vi "File Action V1.vi"(0 "Action":string, 2 "Mode":u16(ring) items=["Read", "Write"], 7 "Image Acquisition Parameters":T2={"Scan Type"=enum."Sample Scanning", "Scan Mode"=enum."XY", "Fast Axis Frequency (Hz)"=100.0, "Image Format"=128, "Line Accumulations"=1, "Frames Per Capture"=1, "Frames Accumulations"=1, "Image Dimension (um)"=[], "Number of Z Steps"=1, "Z Steps Size (um)"=1.0, "Pixel Size (nm)"=[], "Customized Image Format"=[]} {"Z Steps Size (um)" min=0.0; "Number of Z Steps" min=1; "Frames Accumulations" min=1; "Frames Per Capture" min=1; "Line Accumulations" min=1; "Image Format" items=["64 x 64"=64, "128 x 128"=128, "256 x 256"=256, "512 x 512"=512, "1024 x 1024"=1024, "2048 x 2048"=2048, "Customized..."=0]}, 9 "Manual Controls In":T1={"Galvo 1 Position (I16)"=-280, "Galvo 2 Position (I16)"=0, "X Axis Voltage (I16)"=0, "Y Axis Voltage (I16)"=0, "Z Axis Voltage (I16)"=0, "Res Mirror Amp (I16)"=0, "Res Mirror Mute"=FALSE, "Upper Shutter"=FALSE, "Lower Shutter"=FALSE}, 11 "File Path IN":path, 13 "Number of Channels":i32) -> (4 "File Path OUT":path, 8 "File REFs":refnum<file>[](array[refnum]), 15 "Files Open":bool)   [LabVIEW 2014]
uses:
  Type Defs/Image Acquisition Parameters.ctl
  Manual Controls V2.ctl
panel:
  # "Length"
  # "Height"
  # "XY"
  # "Z"
  # "Length"
  # "Height"
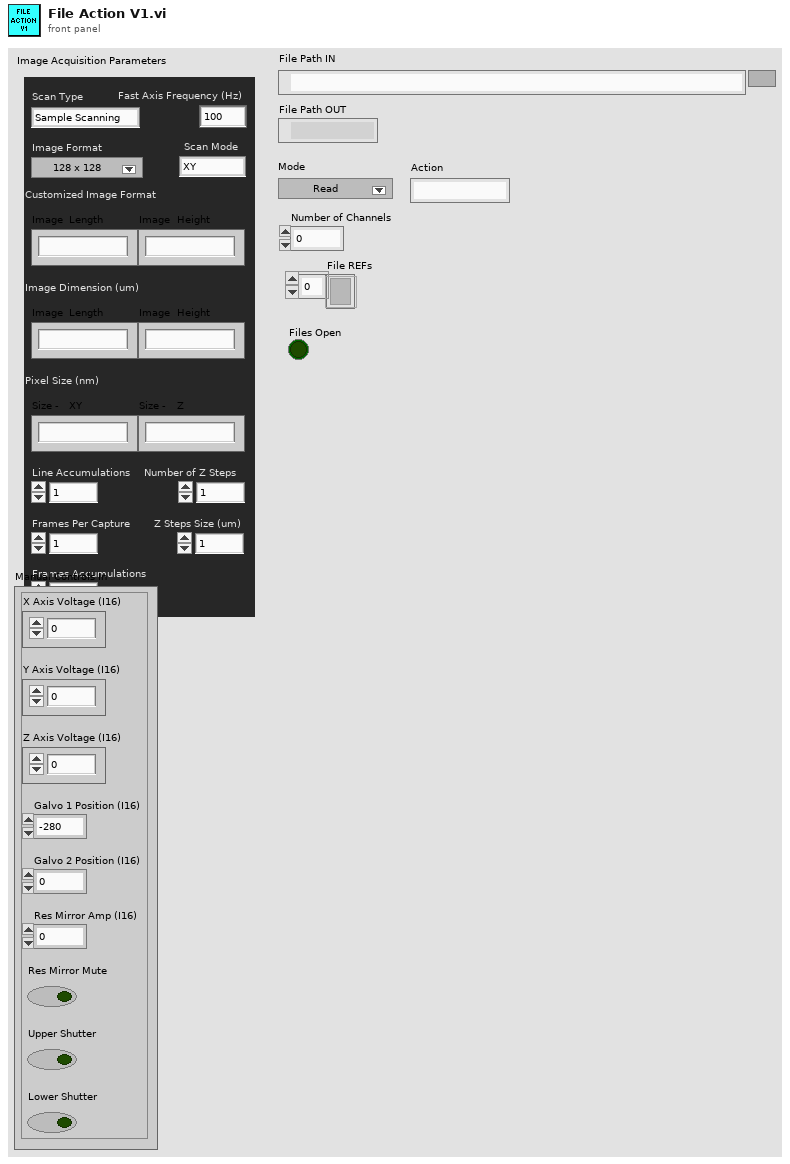
[diagram p1: front panel]
types:
  T1 = typedef "Manual Controls V2.ctl" = cluster{"Galvo 1 Position (I16)":i16, "Galvo 2 Position (I16)":i16, "X Axis Voltage (I16)":i16, "Y Axis Voltage (I16)":i16, "Z Axis Voltage (I16)":i16, "Res Mirror Amp (I16)":i16, "Res Mirror Mute":bool, "Upper Shutter":bool, "Lower Shutter":bool}
  T2 = typedef "Image Acquisition Parameters.ctl" = cluster{"Scan Type":enum16{"Sample Scanning", "Beam Scanning"}, "Scan Mode":enum16{"XY", "XZ", "YZ", "XYZ"}, "Fast Axis Frequency (Hz)":dbl, "Image Format":u16, "Line Accumulations":u16, "Frames Per Capture":u16, "Frames Accumulations":u16, "Image Dimension (um)":dbl[], "Number of Z Steps":u16, "Z Steps Size (um)":dbl, "Pixel Size (nm)":dbl[], "Customized Image Format":dbl[]}
  T3 = cluster{"Z Length (um)":sgl, "Y Length (um)":sgl, "X Length (um)":sgl, "t (s)":sgl}
  T4 = cluster{"Upper Shutter":bool, "Lower Shutter":bool}
  T5 = cluster{"Number of Z Steps":u16, "Image Format":u16, "Image Format":u16, "Frames Per Capture":u16}
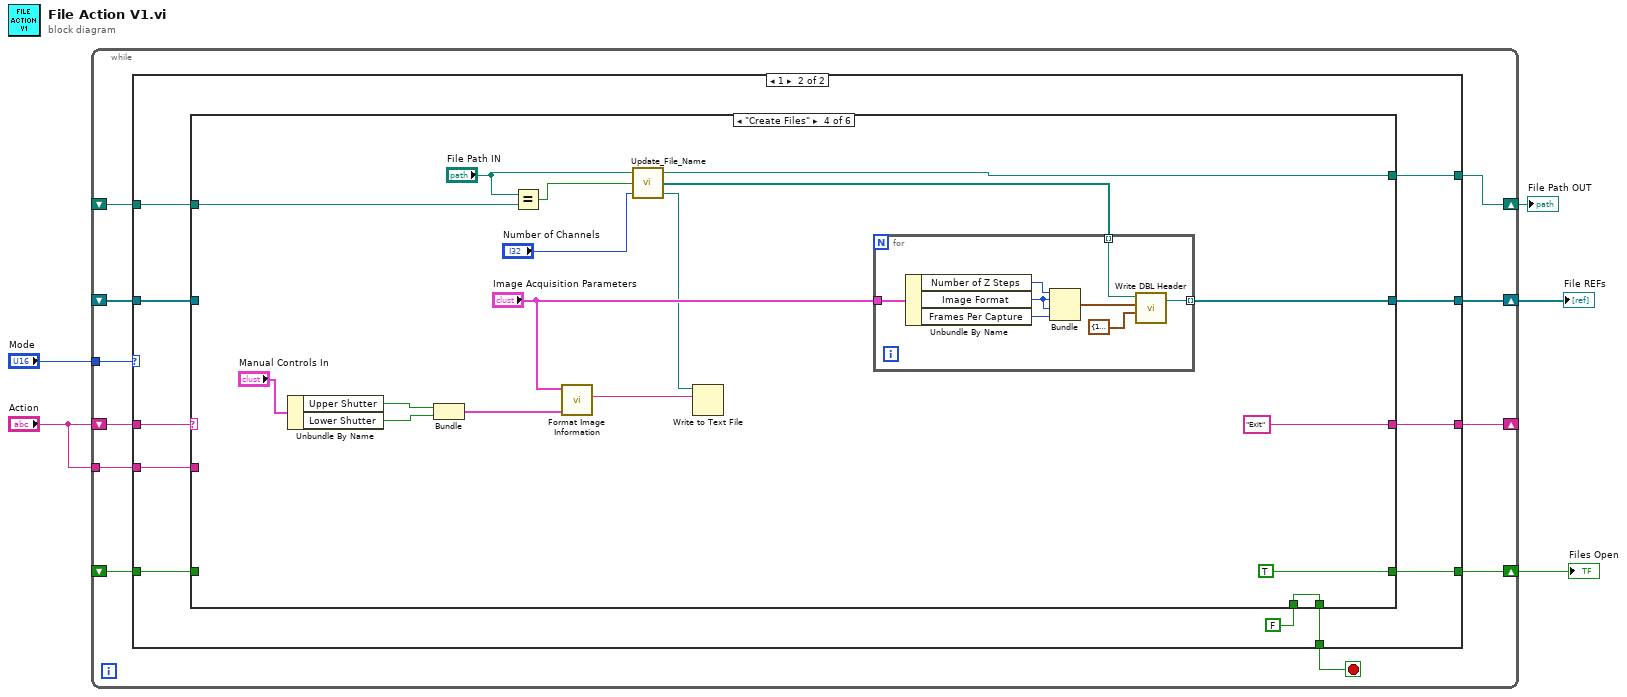
[diagram p0: block diagram]
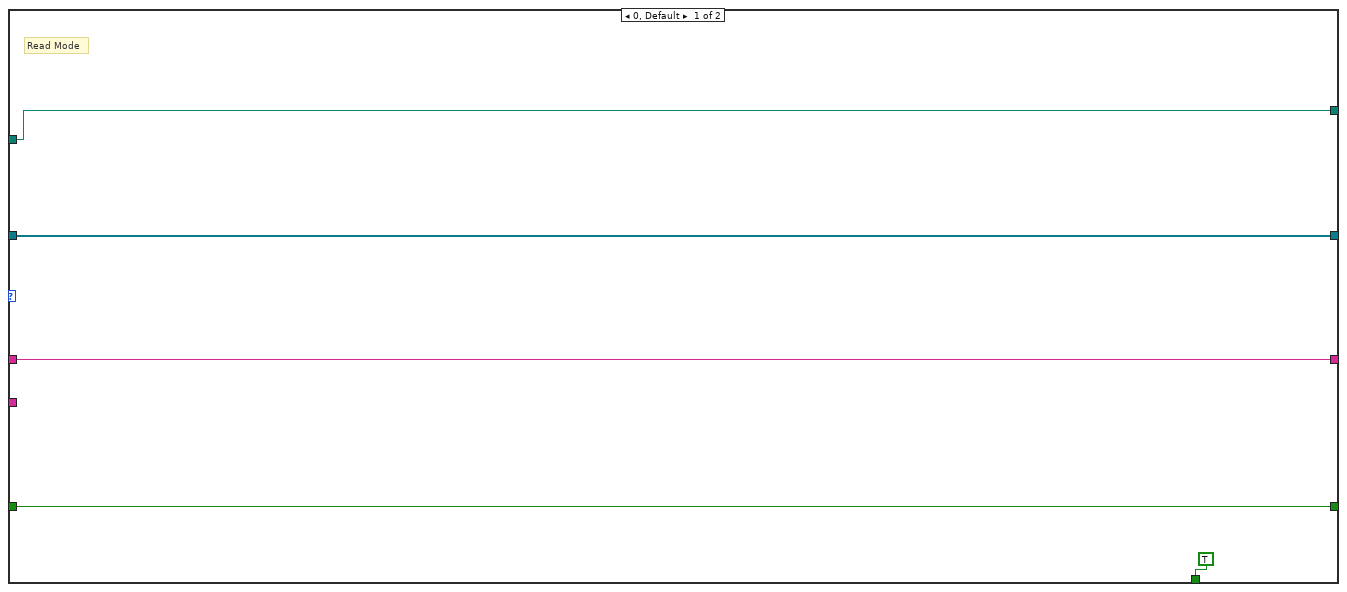
[diagram p2: hidden frame]
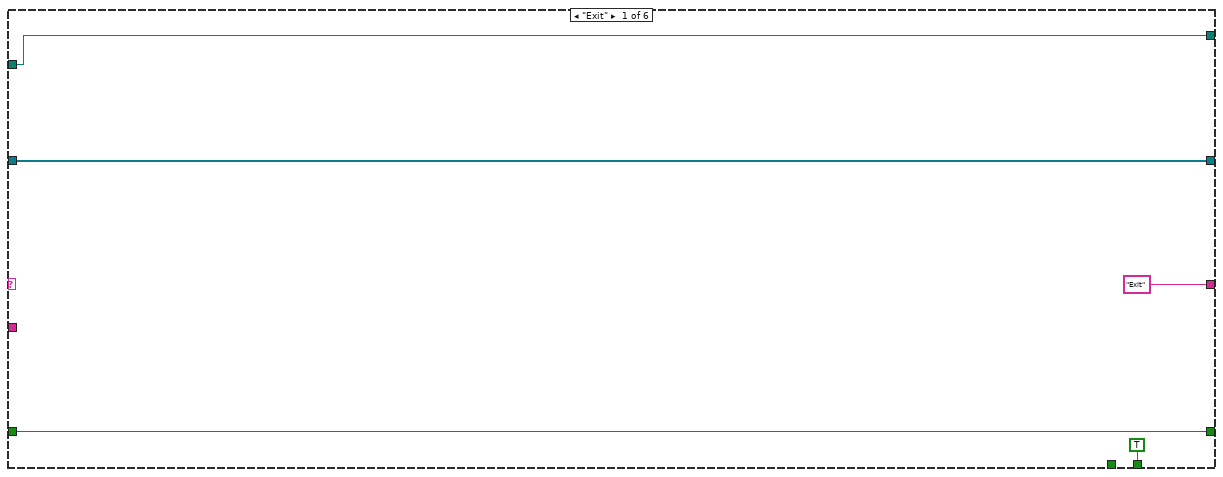
[diagram p3: hidden frame]
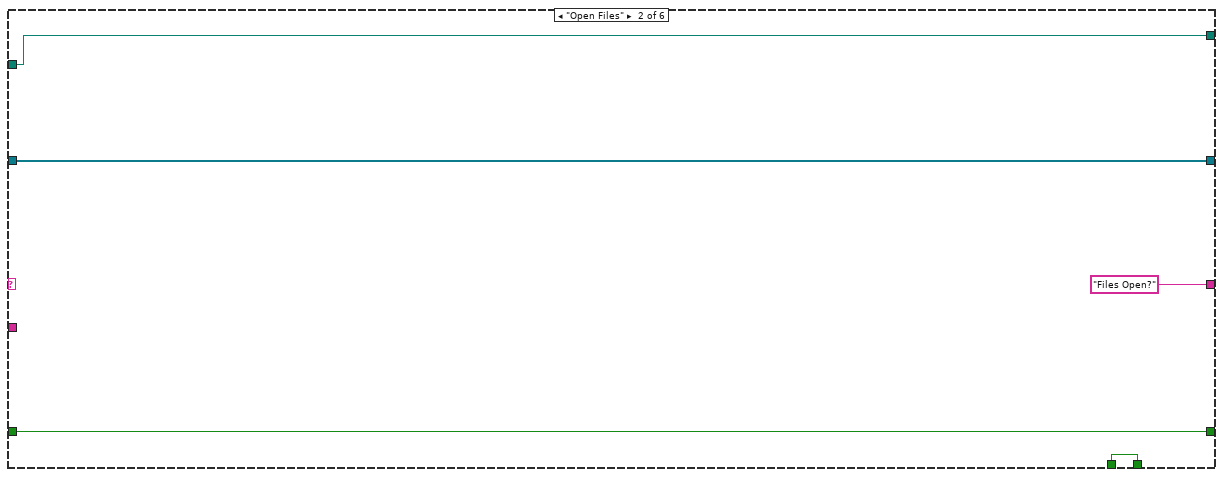
[diagram p4: hidden frame]
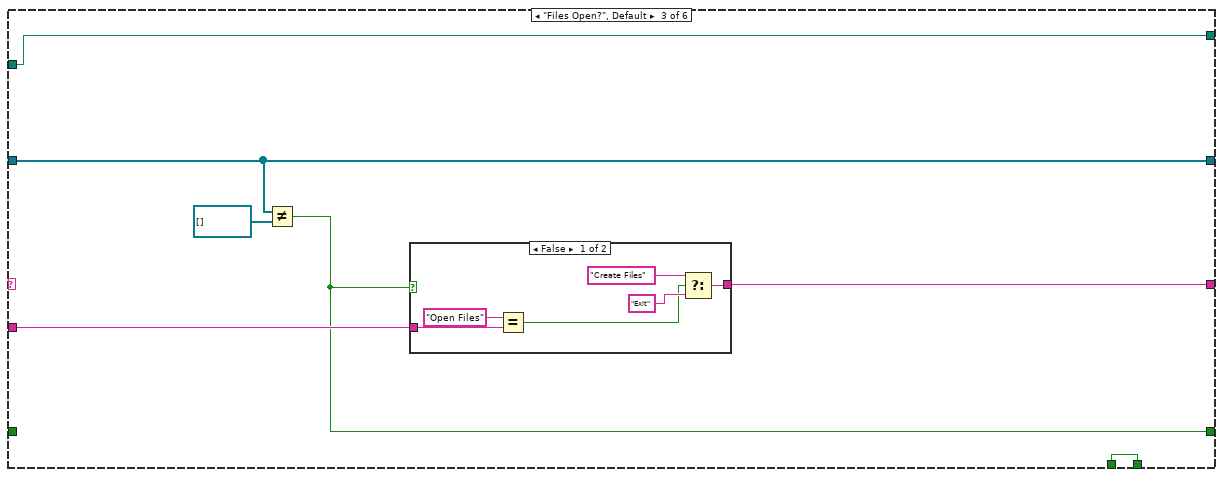
[diagram p5: hidden frame]
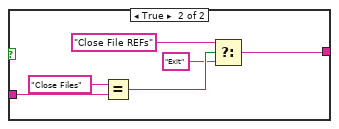
[diagram p6: hidden frame]
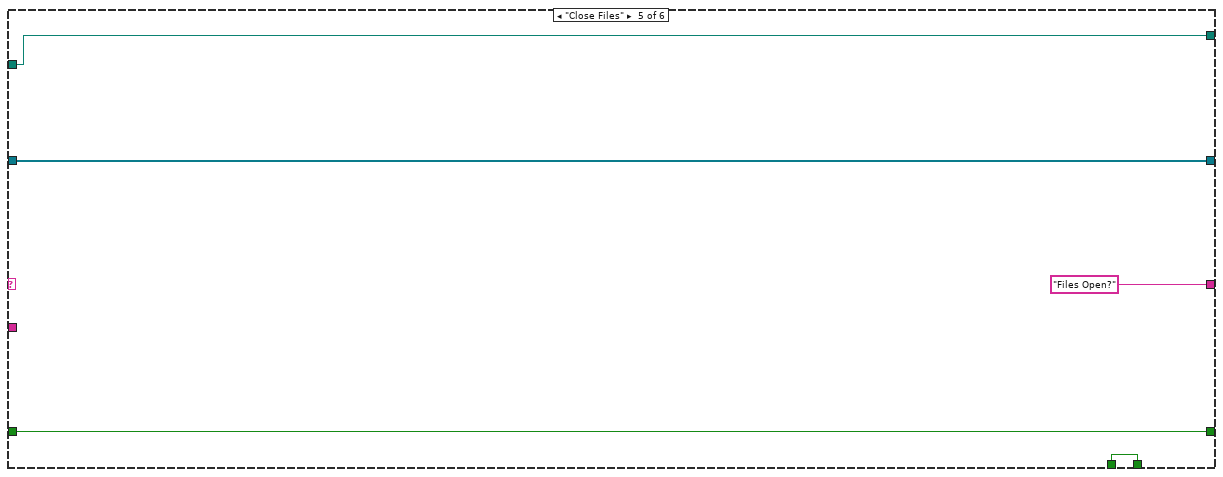
[diagram p7: hidden frame]
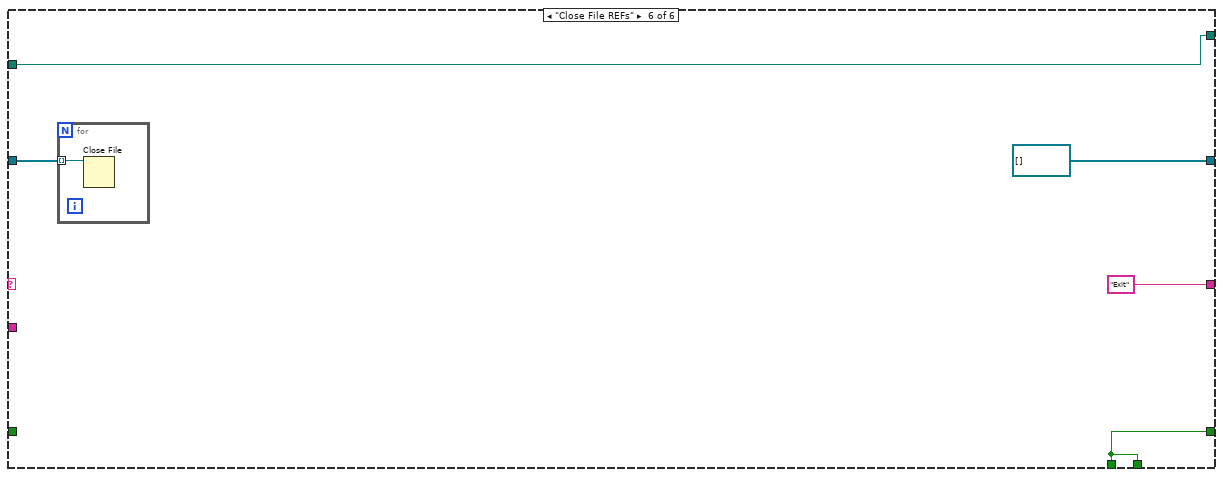
[diagram p8: hidden frame]
diagram:
  n1 = while {
    tunnel: "Mode" -> [w16]
    shift-right: [w15] -> w4
    shift-left: _ -> [w14]
    shift-right: [w12] -> _
    shift-left: "Action" -> [w13]
    tunnel: "Action" -> [w10]
    shift-right: [w9] -> w2
    shift-left: _ -> [w8]
    shift-right: [w7] -> w1
    shift-left: _ -> [w6]
    stop <- w11 stop-if-true
    n2 = case shown="1" w16 {
      tunnel: [w21 w32] -> w15
      tunnel: w14 -> [w21 w30]
      tunnel: w13 -> [w20 w31]
      tunnel: [w20 w29] -> w12
      tunnel: [TRUE w26] -> w11
      tunnel: w10 -> [_ w28]
      tunnel: [w18 w25] -> w9
      tunnel: w8 -> [w18 w24]
      tunnel: [w17 w23] -> w7
      tunnel: w6 -> [w17 w22]
      frame 0, Default {
        # "Read Mode"
      }
      frame 1 {
        n3 = case shown="\"Create Files\"" w31 {
          tunnel: [w35 w42 w48 w68 w91 refnum<file>[] []] -> w32
          tunnel: w30 -> [w35 w42 w48 _ w91 w96]
          tunnel: ["Exit" "Files Open?" w47 "Exit" "Files Open?" "Exit"] -> w29
          tunnel: w28 -> [_ _ w46 _ _ _]
          tunnel: FALSE -> [_ w40 w45 w78 w89 w93]
          tunnel: [TRUE w40 w45 w78 w89 w93] -> w26
          tunnel: [w34 w39 w44 TRUE w88 w93] -> w25
          tunnel: w24 -> [w34 w39 _ _ w88 _]
          tunnel: [w33 w38 w43 w67 w87 w92] -> w23
          tunnel: w22 -> [w33 w38 w43 w75 w87 w92]
          frame "Exit" {
          }
          frame "Open Files" {
          }
          frame "Files Open?", Default {
            n4 = Not Equal?(x=w48, y=refnum<file>[] []) -> (x != y?=w44:bool)
            n5 = case shown="False" w44 {
              tunnel: [w51 w58] -> w47
              tunnel: w46 -> [w55 w60]
              frame False {
                n6 = Equal?(x="Open Files", y=w55) -> (x = y?=w50:bool)
                n7 = Select(t="Create Files", s=w50, f="Exit") -> (s? t:f=w51:string)
              }
              frame True {
                n8 = Equal?(x="Close Files", y=w60) -> (x = y?=w59:bool)
                n9 = Select(t="Close File REFs", s=w59, f="Exit") -> (s? t:f=w58:string)
              }
            }
          }
          frame "Create Files" {
            n10 = Unbundle By Name("Manual Controls In") -> ("Upper Shutter"=w64:bool, "Lower Shutter"=w63:bool)
            n11 = Bundle("Upper Shutter"=w64, "Lower Shutter"=w63) -> (w62:T4)  [unwired: 1 in]
            n12 = Equal?(x="File Path IN", y=w75) -> (x = y?=w70:bool)
            n13 = call "Format Image Information.vi"("Shutters"=w62, "Image Acquisition Parameters"="Image Acquisition Parameters") -> ("Result"=w72:string)  [unwired: 9 in]
            n14 = call "Update_File_Name.vi"("Number of Channels"="Number of Channels", "New File"=w70, "File Path IN"="File Path IN") -> ("Text Image Data Path"=w71:path, "File References"=w69:path[], "File Path OUT"=w67:path)
            n15 = Write to Text File(file (use dialog)=w71, text=w72) -> ()  [unwired: 2 in, 3 out]
            n16 = for {
              tunnel: "Image Acquisition Parameters" -> [w83]
              tunnel: w69 -> [w80] mode=indexing
              tunnel: [w79] -> w68 mode=indexing
              n17 = Unbundle By Name(w83) -> ("Number of Z Steps"=w81:u16, "Image Format"=w85:u16, "Frames Per Capture"=w82:u16)
              n18 = Bundle("Number of Z Steps"=w81, "Image Format"=w85, "Image Format"=w85, "Frames Per Capture"=w82) -> (w84:T5)  [unwired: 1 in]
              n19 = call "Write DBL Header.vi"("Physical Lengths (um)"=T3 {"Z Length (um)"=1.0, "Y Length (um)"=1.0, "X Length (um)"=1.0, "t (s)"=1.0}, "Pixel Lengths"=w84, "File Path IN"=w80) -> ("File Ref OUT"=w79:refnum<file>)  [unwired: 1 in, 1 out]
            }
          }
          frame "Close Files" {
          }
          frame "Close File REFs" {
            n20 = for {
              tunnel: w96 -> [w97] mode=indexing
              n21 = Close File(refnum=w97) -> ()  [unwired: 1 in, 2 out]
            }
          }
        }
      }
    }
  }
  "File REFs" <- w4
  "Files Open" <- w2
  "File Path OUT" <- w1
